vi "ConvertSamples.vi"(8 "ErrorIn":errorcluster, 10 "MeasurementConfig":T5={"Frequency"=100, "Resolution[b]"=16, "AccelFSRange"=enum."+/-2g", "GyroFSRange"=enum."+/-250dps"} {"Resolution[b]" min=4 max=16 step=1; "Frequency" min=1 max=10000000 step=1}, 11 "SamplesIn":T3[](array[typedef])) -> (0 "ErrorOut":errorcluster, 3 "SamplesOut":T1[](array[typedef]))   [LabVIEW 2016]
doc: "Convert raw intertial measurement samples to useful data."
uses:
  MeasurementConfig.ctl
  AccelFSRange.ctl
  GyroFSRange.ctl
  Sample.ctl
  Reading.ctl
  MeasSample.ctl
  MeasReading.ctl
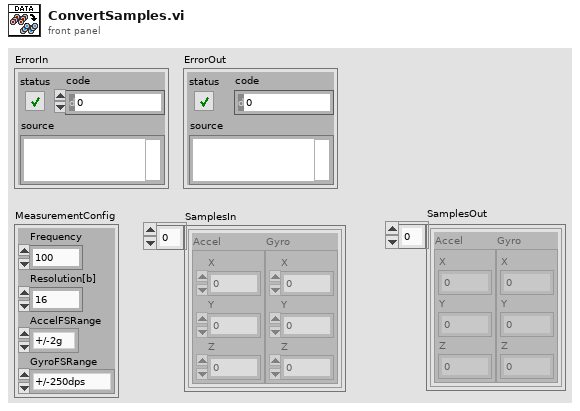
[diagram p1: front panel]
types:
  T1 = typedef "MeasSample.ctl" = cluster{"Accel":T2, "Gyro":T2}
  T2 = typedef "MeasReading.ctl" = cluster{"X":dbl, "Y":dbl, "Z":dbl}
  T3 = typedef "Sample.ctl" = cluster{"Accel":T4, "Gyro":T4}
  T4 = typedef "Reading.ctl" = cluster{"X":i16, "Y":i16, "Z":i16}
  T5 = typedef "MeasurementConfig.ctl" = cluster{"Frequency":u32, "Resolution[b]":u32, "AccelFSRange":T6, "GyroFSRange":T7}
  T6 = typedef "AccelFSRange.ctl" = enum16{"+/-2g", "+/-4g", "+/-8g", "+/-16g"}
  T7 = typedef "GyroFSRange.ctl" = enum16{"+/-250dps", "+/-500dps", "+/-1000dps", "+/-2000dps"}
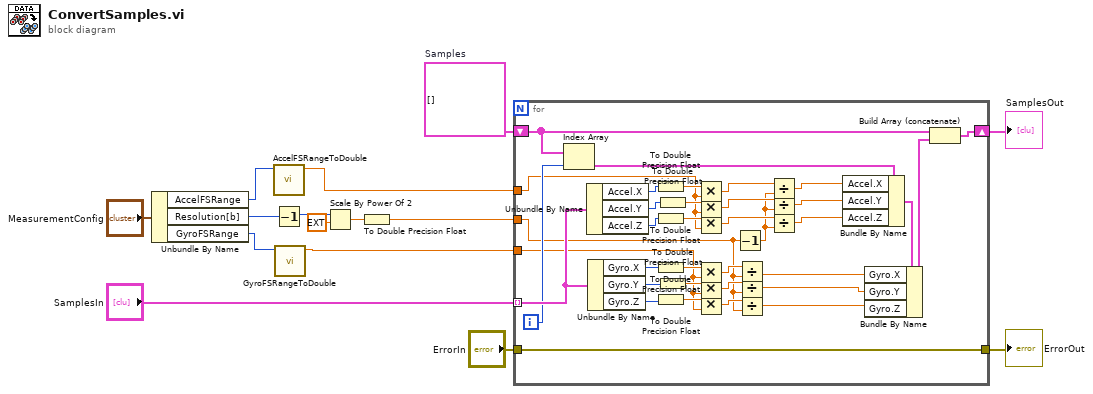
[diagram p0: block diagram]
diagram:
  w9 = T1[] []  # Samples
  n1 = Unbundle By Name("MeasurementConfig") -> ("AccelFSRange"=w4:T6, "Resolution[b]"=w13:u32, "GyroFSRange"=w2:T7)
  n2 = call "AccelFSRangeToDouble.vi"("AccelFSRange"=w4) -> ("Double"=w3:dbl)  [unwired: 10 in]
  n3 = Decrement(x=w13) -> (x-1=w12:u32)
  n4 = call "GyroFSRangeToDouble.vi"("GyroFSRange"=w2) -> ("Double"=w1:dbl)  [unwired: 10 in]
  n5 = Scale By Power Of 2(n=w12, x=ext 1.0) -> (x*2^n=w10:ext)
  n6 = To Double Precision Float(number=w10) -> (double precision float=w8:dbl)
  n7 = for {
    tunnel: "SamplesIn" -> [w51] mode=indexing
    tunnel: w3 -> [w40]
    tunnel: w8 -> [w26]
    tunnel: w1 -> [w33]
    shift-right: [w50] -> w7
    shift-left: w9 -> [w49]
    tunnel: "ErrorIn" -> [w17]
    tunnel: [w17] -> w5
    i -> [w48]
    n8 = Index Array(array=w49, index=w48) -> (element=w47:T1)
    n9 = Unbundle By Name(w51) -> ("Accel.X"=w44:i16, "Accel.Y"=w46:i16, "Accel.Z"=w45:i16)
    n10 = Unbundle By Name(w51) -> ("Gyro.X"=w36:i16, "Gyro.Y"=w35:i16, "Gyro.Z"=w34:i16)
    n11 = To Double Precision Float(number=w44) -> (double precision float=w43:dbl)
    n12 = To Double Precision Float(number=w45) -> (double precision float=w41:dbl)
    n13 = To Double Precision Float(number=w36) -> (double precision float=w37:dbl)
    n14 = To Double Precision Float(number=w34) -> (double precision float=w39:dbl)
    n15 = To Double Precision Float(number=w46) -> (double precision float=w42:dbl)
    n16 = To Double Precision Float(number=w35) -> (double precision float=w38:dbl)
    n17 = Multiply(x=w43, y=w40) -> (x*y=w27:dbl)
    n18 = Multiply(x=w42, y=w40) -> (x*y=w29:dbl)
    n19 = Multiply(x=w41, y=w40) -> (x*y=w28:dbl)
    n20 = Multiply(x=w37, y=w33) -> (x*y=w31:dbl)
    n21 = Multiply(x=w38, y=w33) -> (x*y=w30:dbl)
    n22 = Multiply(x=w39, y=w33) -> (x*y=w32:dbl)
    n23 = Decrement(x=w26) -> (x-1=w16:dbl)
    n24 = Divide(x=w31, y=w26) -> (x/y=w22:dbl)
    n25 = Divide(x=w30, y=w26) -> (x/y=w21:dbl)
    n26 = Divide(x=w32, y=w26) -> (x/y=w20:dbl)
    n27 = Divide(x=w27, y=w16) -> (x/y=w25:dbl)
    n28 = Divide(x=w29, y=w16) -> (x/y=w24:dbl)
    n29 = Divide(x=w28, y=w16) -> (x/y=w23:dbl)
    n30 = Bundle By Name(cluster=w47, "Accel.X"=w25, "Accel.Y"=w24, "Accel.Z"=w23) -> (w19:T1)
    n31 = Bundle By Name(cluster=w19, "Gyro.X"=w22, "Gyro.Y"=w21, "Gyro.Z"=w20) -> (w18:T1)
    n32 = Build Array (concatenate)(w49, w18) -> (w50:T1[])
  }
  "ErrorOut" <- w5
  "SamplesOut" <- w7
